vi "Draw Range Border.vi"(4 "Marker Options":T2={"Color"=16723218, "pen"={"Width"=2, "Style"=enum."Solid"}, "font"={"Font Name"="Arial", "Size"=16, "Strikeout?"=FALSE, "Italic?"=FALSE, "Underline?"=FALSE, "Outline?"=FALSE, "Shadow?"=FALSE, "Bold?"=FALSE, "FontColor"=0}, "caption"=""}, 6 "Type":T1, 7 "picture":picture, 9 "end Coords":T3, 10 "Plot Bounds":T4, 11 "Start Coords":T3) -> (5 "new picture":picture)   [LabVIEW 2015]
uses:
  <vilib>/Utility/miscctls.llb/LVRectTypeDef.ctl
  <vilib>/Utility/miscctls.llb/LVPoint32TypeDef.ctl
  controls/MarkerOptions.ctl
  controls/markerType.ctl
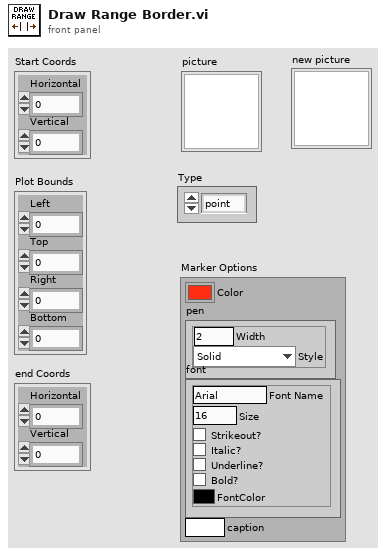
[diagram p1: front panel]
types:
  T1 = typedef "markerType.ctl" = enum16{"point", "arrow", "horiz", "vert", "vert range", "horiz range", "box"}
  T2 = typedef "MarkerOptions.ctl" = cluster{"Color":u32, "pen":cluster{"Width":u16, "Style":enum32{"Solid", "Dash", "Dot", "DashDot", "DashDotDot"}}, "font":cluster{"Font Name":string, "Size":i16, "Strikeout?":bool, "Italic?":bool, "Underline?":bool, "Outline?":bool, "Shadow?":bool, "Bold?":bool, "FontColor":u32}, "caption":string}
  T3 = typedef "LVPoint32TypeDef.ctl" = cluster{"Horizontal":i32, "Vertical":i32}
  T4 = typedef "LVRectTypeDef.ctl" = cluster{"Left":i16, "Top":i16, "Right":i16, "Bottom":i16}
  T5 = cluster{"Width":u16, "Style":enum32{"Solid", "Dash", "Dot", "DashDot", "DashDotDot"}}
  T6 = cluster{"left":i16, "top":i16, "right":i16, "bottom":i16}
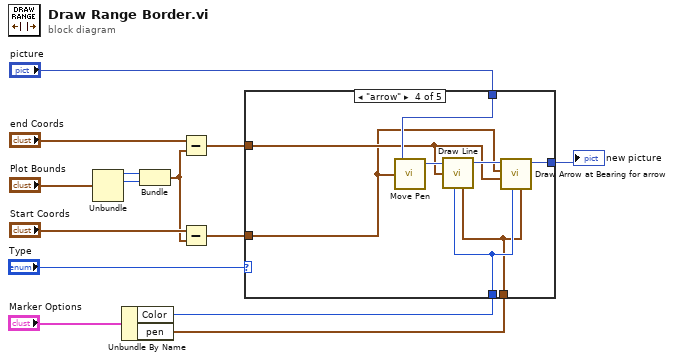
[diagram p0: block diagram]
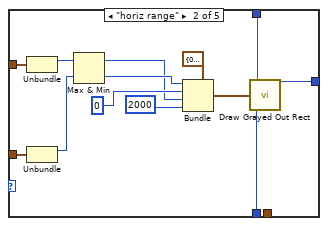
[diagram p3: hidden frame]
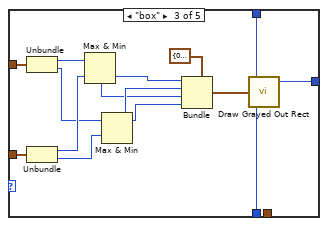
[diagram p4: hidden frame]
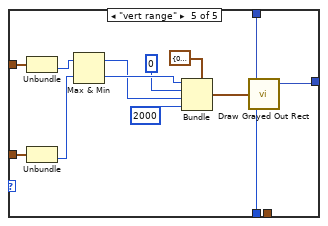
[diagram p5: hidden frame]
diagram:
  n1 = Unbundle("Plot Bounds") -> ("Left"=w14:i16, "Top"=w11:i16)  [unwired: 2 out]
  n2 = Unbundle By Name("Marker Options") -> ("Color"=w3:u32, "pen"=w1:T5)
  n3 = Bundle("Left"=w14, "Top"=w11) -> (w7:cluster{"Left":i16, "Top":i16})  [unwired: 1 in]
  n4 = Subtract(x="end Coords", y=w7) -> (x-y=w10:T3)
  n5 = Subtract(x="Start Coords", y=w7) -> (x-y=w9:T3)
  n6 = case shown="\"arrow\"" "Type" {
    tunnel: w10 -> [_ w26 w41 w47 w64]
    tunnel: w9 -> [_ w25 w40 w45 w63]
    tunnel: [w15 w22 w32 w48 w58] -> w4
    tunnel: w3 -> [_ w20 w31 w46 w56]
    tunnel: "picture" -> [w15 w21 w30 w51 w57]
    tunnel: w1 -> [_ _ _ w44 _]
    frame Default {
    }
    frame "horiz range" {
      n7 = Unbundle(w26) -> ("Horizontal"=w27:i32)  [unwired: 1 out]
      n8 = Unbundle(w25) -> ("Horizontal"=w28:i32)  [unwired: 1 out]
      n9 = Max & Min(x=w27, y=w28) -> (max(x,y)=w16:i32, min(x,y)=w17:i32)
      n10 = Bundle(cluster=T6 {"left"=0, "top"=0, "right"=0, "bottom"=0} ("rect"), "left"=w17, "top"=i16 0, "right"=w16, "bottom"=i16 2000 ("top")) -> (w24:T6)
      n11 = call <vilib>:"Draw Grayed Out Rect.vi"("color(black)"=w20, "rect"=w24, "picture"=w21) -> ("new picture"=w22:picture)  [unwired: 2 in]
    }
    frame "box" {
      n12 = Unbundle(w41) -> ("Horizontal"=w42:i32, "Vertical"=w38:i32)
      n13 = Unbundle(w40) -> ("Horizontal"=w43:i32, "Vertical"=w39:i32)
      n14 = Max & Min(x=w42, y=w43) -> (max(x,y)=w35:i32, min(x,y)=w37:i32)
      n15 = Max & Min(x=w38, y=w39) -> (max(x,y)=w34:i32, min(x,y)=w36:i32)
      n16 = Bundle(cluster=T6 {"left"=0, "top"=0, "right"=0, "bottom"=0} ("rect"), "left"=w37, "top"=w36, "right"=w35, "bottom"=w34) -> (w33:T6)
      n17 = call <vilib>:"Draw Grayed Out Rect.vi"("color(black)"=w31, "rect"=w33, "picture"=w30) -> ("new picture"=w32:picture)  [unwired: 2 in]
    }
    frame "arrow" {
      n18 = call <vilib>:"Move Pen.vi"("new position"=w45, "picture"=w51) -> ("new picture"=w50:picture)  [unwired: 3 in]
      n19 = call <vilib>:"Draw Line.vi"("picture"=w50, "end point"=w47, "color(black)"=w46, "pen"=w44) -> ("new picture"=w49:picture)  [unwired: 5 in]
      n20 = call "Draw Arrow at Bearing for arrow.vi"("pen"=w44, "color(black)"=w46, "P2"=w47, "P1"=w45, "new picture in"=w49) -> ("new picture out"=w48:picture)  [unwired: 6 in]
    }
    frame "vert range" {
      n21 = Unbundle(w64) -> ("Vertical"=w62:i32)  [unwired: 1 out]
      n22 = Unbundle(w63) -> ("Vertical"=w61:i32)  [unwired: 1 out]
      n23 = Max & Min(x=w62, y=w61) -> (max(x,y)=w52:i32, min(x,y)=w55:i32)
      n24 = Bundle(cluster=T6 {"left"=0, "top"=0, "right"=0, "bottom"=0} ("rect"), "left"=w55, "top"=i16 0, "right"=w52, "bottom"=i16 2000 ("top")) -> (w60:T6)
      n25 = call <vilib>:"Draw Grayed Out Rect.vi"("color(black)"=w56, "rect"=w60, "picture"=w57) -> ("new picture"=w58:picture)  [unwired: 2 in]
    }
  }
  "new picture" <- w4
